vi "Set-UI-state.vi"(6 "State":T1, 8 "error in":errorcluster, 10 "Data ref. in":refnum<data-value>, 11 "UI ref. in":refnum<data-value>) -> (0 "error IO":errorcluster, 2 "Data ref.":refnum<data-value>, 3 "UI ref.":refnum<data-value>)   [LabVIEW 2013, in "CameraVision.lvlib" / "CV-UI.lvclass"]
doc: "This function deletes the data from the various GUI graphs and displays. This avoids interference with data from a previous acquisition."
uses:
  CV-UI.lvclass
  Main/Application-states.ctl
  Main/CV-Main.lvclass
  Control-names.ctl
  Main/Enqueue-modes.ctl
  Main/Main-actions.ctl
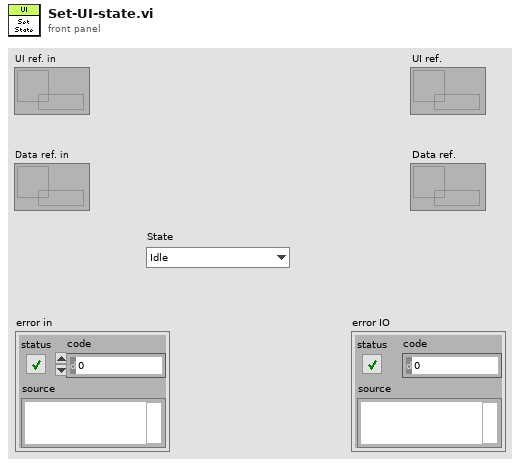
[diagram p1: front panel]
types:
  T1 = typedef "CameraVision.lvlib/CV-Main.lvclass/Application-states.ctl" = enum16{"Idle", "Initialized", "Configured", "Activated", "Started", "Stopped", "Reset", "Error", "Exited"}
  T2 = typedef "CameraVision.lvlib/CV-Main.lvclass/Enqueue-modes.ctl" = enum16{"Default", "Priority", "Flush"}
  T3 = typedef "CameraVision.lvlib/CV-UI.lvclass/Control-names.ctl" = enum16{"Start acquisition", "Activate", "Stop acquisition", "Settings type", "Load settings", "Save settings", "Import images", "Camera selector", "Image type selector", "Batch browser", "Image refresh", "Parameter tabs", "Displays", "Processing tabs", "Processing selector", "Map characteristic", "Show info", "Manual trigger"}
  T4 = typedef "CameraVision.lvlib/CV-Main.lvclass/Main-actions.ctl" = enum16{"Idle", "Initialize", "Load defaults", "Update settings", "Check settings", "Save settings", "Save settings with dialog", "Load settings", "Load data", "Activate", "Start", "Wait for start signal", "Acquire & process", "Iterate", "Stop", "Refresh display", "Refresh status", "View camera settings", "View grabber settings", "Exit"}
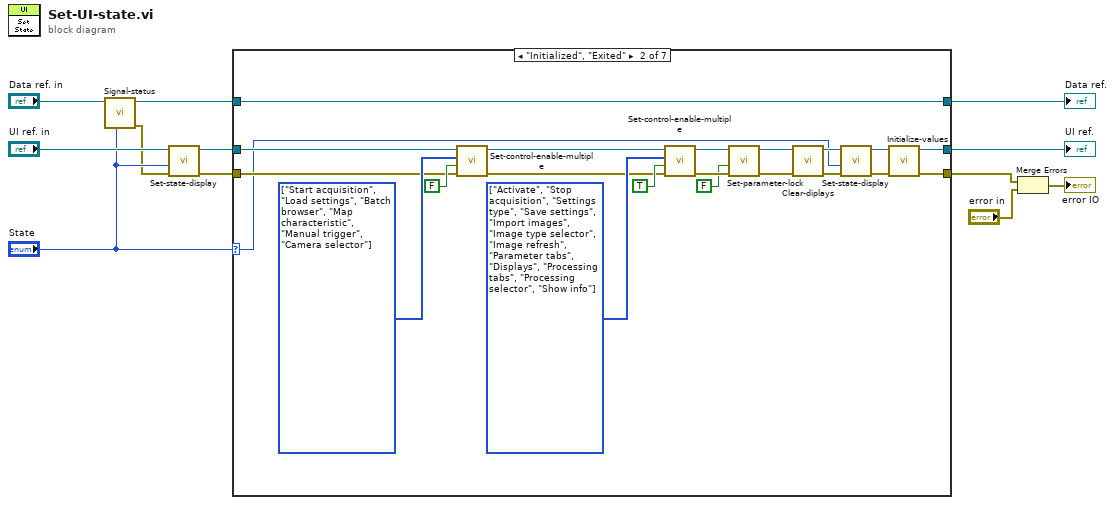
[diagram p0: block diagram]
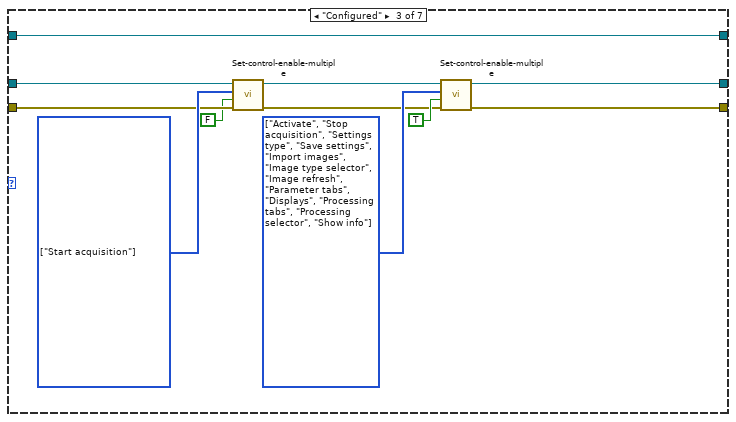
[diagram p3: hidden frame]
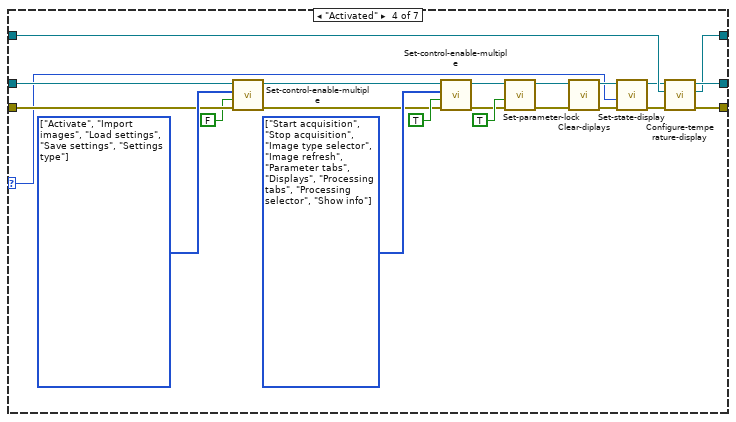
[diagram p4: hidden frame]
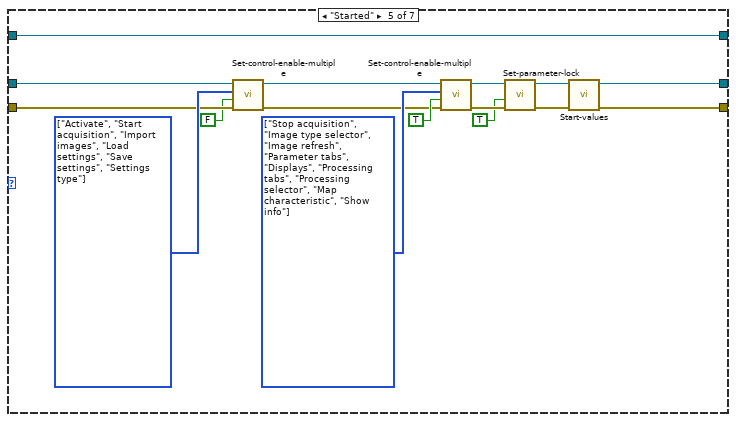
[diagram p5: hidden frame]
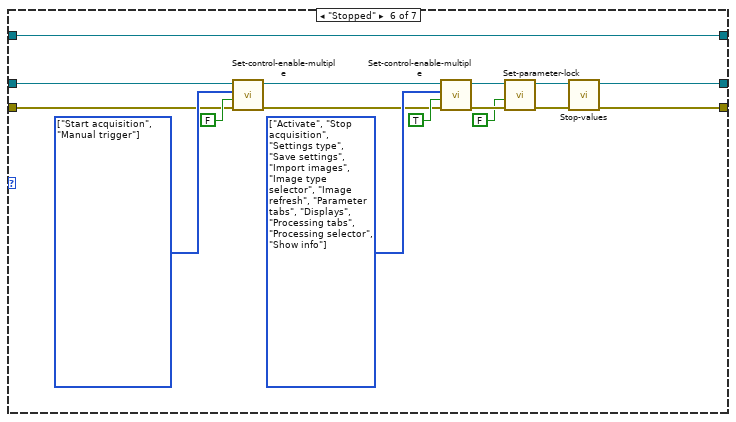
[diagram p6: hidden frame]
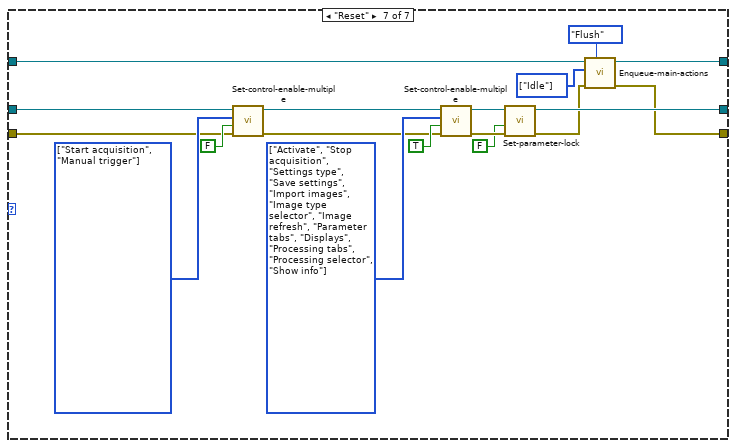
[diagram p7: hidden frame]
diagram:
  n1 = call "Signal-status.vi"("State"="State", "Data ref. in"="Data ref. in") -> ("error out"=w3:errorcluster, "Data ref."=w6:refnum<data-value>)  [unwired: 8 in]
  n2 = call "Set-state-display.vi"("error in"=w3, "State"="State", "UI ref. in"="UI ref. in") -> ("error IO"=w4:errorcluster, "UI ref."=w5:refnum<data-value>)  [unwired: 7 in]
  n3 = case shown="\"Initialized\", \"Exited\"" "State" {
    selector: "State" -> [_ w16 _ w48 _ _ _]
    tunnel: w4 -> [w14 w22 w45 w67 w83 w86 w108]
    tunnel: w5 -> [w15 w35 w46 w68 w84 w100 w118]
    tunnel: [w15 w23 w38 w56 w73 w91 w107] -> w10
    tunnel: [w14 w24 w39 w53 w74 w88 w104] -> w12
    tunnel: w6 -> [w13 w21 w37 w55 w70 w87 w109]
    tunnel: [w13 w21 w37 w54 w70 w87 w106] -> w7
    frame Default {
    }
    frame "Initialized", "Exited" {
      w33 = T3[] [enum."Activate", enum."Stop acquisition", enum."Settings type", enum."Save settings", enum."Import images", enum."Image type selector", enum."Image refresh", enum."Parameter tabs", enum."Displays", enum."Processing tabs", enum."Processing selector", enum."Show info"] items=["Start acquisition", "Activate", "Stop acquisition", "Settings type", "Load settings", "Save settings", "Import images", "Camera selector", "Image type selector", "Batch browser", "Image refresh", "Parameter tabs", "Displays", "Processing tabs", "Processing selector", "Map characteristic", "Show info", "Manual trigger"] ("Control names")
      w36 = T3[] [enum."Start acquisition", enum."Load settings", enum."Batch browser", enum."Map characteristic", enum."Manual trigger", enum."Camera selector"] items=["Start acquisition", "Activate", "Stop acquisition", "Settings type", "Load settings", "Save settings", "Import images", "Camera selector", "Image type selector", "Batch browser", "Image refresh", "Parameter tabs", "Displays", "Processing tabs", "Processing selector", "Map characteristic", "Show info", "Manual trigger"] ("Control names")
      n4 = call "Set-control-enable-multiple.vi"("error in (no error)"=w22, "Enable?"=FALSE, "Control names"=w36, "UI ref. in"=w35) -> ("error out"=w31:errorcluster, "UI ref."=w30:refnum<data-value>)  [unwired: 6 in]
      n5 = call "Set-control-enable-multiple.vi"("error in (no error)"=w31, "Enable?"=TRUE, "Control names"=w33, "UI ref. in"=w30) -> ("error out"=w28:errorcluster, "UI ref."=w29:refnum<data-value>)  [unwired: 6 in]
      n6 = call "Set-parameter-lock.vi"("error in (no error)"=w28, "Lock?"=FALSE, "UI ref. in"=w29) -> ("error out"=w25:errorcluster, "UI ref."=w26:refnum<data-value>)  [unwired: 7 in]
      n7 = call "Clear-diplays.vi"("error in"=w25, "UI ref. in"=w26) -> ("error IO"=w17:errorcluster, "UI ref."=w20:refnum<data-value>)  [unwired: 8 in]
      n8 = call "Set-state-display.vi"("error in"=w17, "State"=w16, "UI ref. in"=w20) -> ("error IO"=w18:errorcluster, "UI ref."=w19:refnum<data-value>)  [unwired: 7 in]
      n9 = call "Initialize-values.vi"("error in"=w18, "UI ref. in"=w19) -> ("error IO"=w24:errorcluster, "UI ref."=w23:refnum<data-value>)  [unwired: 8 in]
    }
    frame "Configured" {
      w43 = T3[] [enum."Activate", enum."Stop acquisition", enum."Settings type", enum."Save settings", enum."Import images", enum."Image type selector", enum."Image refresh", enum."Parameter tabs", enum."Displays", enum."Processing tabs", enum."Processing selector", enum."Show info"] items=["Start acquisition", "Activate", "Stop acquisition", "Settings type", "Load settings", "Save settings", "Import images", "Camera selector", "Image type selector", "Batch browser", "Image refresh", "Parameter tabs", "Displays", "Processing tabs", "Processing selector", "Map characteristic", "Show info", "Manual trigger"] ("Control names")
      w47 = T3[] [enum."Start acquisition"] items=["Start acquisition", "Activate", "Stop acquisition", "Settings type", "Load settings", "Save settings", "Import images", "Camera selector", "Image type selector", "Batch browser", "Image refresh", "Parameter tabs", "Displays", "Processing tabs", "Processing selector", "Map characteristic", "Show info", "Manual trigger"] ("Control names")
      n10 = call "Set-control-enable-multiple.vi"("error in (no error)"=w45, "Enable?"=FALSE, "Control names"=w47, "UI ref. in"=w46) -> ("error out"=w41:errorcluster, "UI ref."=w40:refnum<data-value>)  [unwired: 6 in]
      n11 = call "Set-control-enable-multiple.vi"("error in (no error)"=w41, "Enable?"=TRUE, "Control names"=w43, "UI ref. in"=w40) -> ("error out"=w39:errorcluster, "UI ref."=w38:refnum<data-value>)  [unwired: 6 in]
    }
    frame "Activated" {
      w65 = T3[] [enum."Start acquisition", enum."Stop acquisition", enum."Image type selector", enum."Image refresh", enum."Parameter tabs", enum."Displays", enum."Processing tabs", enum."Processing selector", enum."Show info"] items=["Start acquisition", "Activate", "Stop acquisition", "Settings type", "Load settings", "Save settings", "Import images", "Camera selector", "Image type selector", "Batch browser", "Image refresh", "Parameter tabs", "Displays", "Processing tabs", "Processing selector", "Map characteristic", "Show info", "Manual trigger"] ("Control names")
      w69 = T3[] [enum."Activate", enum."Import images", enum."Load settings", enum."Save settings", enum."Settings type"] items=["Start acquisition", "Activate", "Stop acquisition", "Settings type", "Load settings", "Save settings", "Import images", "Camera selector", "Image type selector", "Batch browser", "Image refresh", "Parameter tabs", "Displays", "Processing tabs", "Processing selector", "Map characteristic", "Show info", "Manual trigger"] ("Control names")
      n12 = call "Set-control-enable-multiple.vi"("error in (no error)"=w67, "Enable?"=FALSE, "Control names"=w69, "UI ref. in"=w68) -> ("error out"=w63:errorcluster, "UI ref."=w62:refnum<data-value>)  [unwired: 6 in]
      n13 = call "Set-control-enable-multiple.vi"("error in (no error)"=w63, "Enable?"=TRUE, "Control names"=w65, "UI ref. in"=w62) -> ("error out"=w59:errorcluster, "UI ref."=w60:refnum<data-value>)  [unwired: 6 in]
      n14 = call "Set-parameter-lock.vi"("error in (no error)"=w59, "Lock?"=TRUE, "UI ref. in"=w60) -> ("error out"=w58:errorcluster, "UI ref."=w57:refnum<data-value>)  [unwired: 7 in]
      n15 = call "Clear-diplays.vi"("error in"=w58, "UI ref. in"=w57) -> ("error IO"=w49:errorcluster, "UI ref."=w52:refnum<data-value>)  [unwired: 8 in]
      n16 = call "Set-state-display.vi"("error in"=w49, "State"=w48, "UI ref. in"=w52) -> ("error IO"=w50:errorcluster, "UI ref."=w51:refnum<data-value>)  [unwired: 7 in]
      n17 = call "Configure-temperature-display.vi"("error in"=w50, "Data ref. in"=w55, "UI ref. in"=w51) -> ("error IO"=w53:errorcluster, "Data ref."=w54:refnum<data-value>, "UI ref."=w56:refnum<data-value>)  [unwired: 6 in]
    }
    frame "Started" {
      w81 = T3[] [enum."Stop acquisition", enum."Image type selector", enum."Image refresh", enum."Parameter tabs", enum."Displays", enum."Processing tabs", enum."Processing selector", enum."Map characteristic", enum."Show info"] items=["Start acquisition", "Activate", "Stop acquisition", "Settings type", "Load settings", "Save settings", "Import images", "Camera selector", "Image type selector", "Batch browser", "Image refresh", "Parameter tabs", "Displays", "Processing tabs", "Processing selector", "Map characteristic", "Show info", "Manual trigger"] ("Control names")
      w85 = T3[] [enum."Activate", enum."Start acquisition", enum."Import images", enum."Load settings", enum."Save settings", enum."Settings type"] items=["Start acquisition", "Activate", "Stop acquisition", "Settings type", "Load settings", "Save settings", "Import images", "Camera selector", "Image type selector", "Batch browser", "Image refresh", "Parameter tabs", "Displays", "Processing tabs", "Processing selector", "Map characteristic", "Show info", "Manual trigger"] ("Control names")
      n18 = call "Set-control-enable-multiple.vi"("error in (no error)"=w83, "Enable?"=FALSE, "Control names"=w85, "UI ref. in"=w84) -> ("error out"=w79:errorcluster, "UI ref."=w78:refnum<data-value>)  [unwired: 6 in]
      n19 = call "Set-control-enable-multiple.vi"("error in (no error)"=w79, "Enable?"=TRUE, "Control names"=w81, "UI ref. in"=w78) -> ("error out"=w76:errorcluster, "UI ref."=w77:refnum<data-value>)  [unwired: 6 in]
      n20 = call "Set-parameter-lock.vi"("error in (no error)"=w76, "Lock?"=TRUE, "UI ref. in"=w77) -> ("error out"=w71:errorcluster, "UI ref."=w72:refnum<data-value>)  [unwired: 7 in]
      n21 = call "Start-values.vi"("error in"=w71, "UI ref. in"=w72) -> ("error IO"=w74:errorcluster, "UI ref."=w73:refnum<data-value>)  [unwired: 8 in]
    }
    frame "Stopped" {
      w98 = T3[] [enum."Activate", enum."Stop acquisition", enum."Settings type", enum."Save settings", enum."Import images", enum."Image type selector", enum."Image refresh", enum."Parameter tabs", enum."Displays", enum."Processing tabs", enum."Processing selector", enum."Show info"] items=["Start acquisition", "Activate", "Stop acquisition", "Settings type", "Load settings", "Save settings", "Import images", "Camera selector", "Image type selector", "Batch browser", "Image refresh", "Parameter tabs", "Displays", "Processing tabs", "Processing selector", "Map characteristic", "Show info", "Manual trigger"] ("Control names")
      w101 = T3[] [enum."Start acquisition", enum."Manual trigger"] items=["Start acquisition", "Activate", "Stop acquisition", "Settings type", "Load settings", "Save settings", "Import images", "Camera selector", "Image type selector", "Batch browser", "Image refresh", "Parameter tabs", "Displays", "Processing tabs", "Processing selector", "Map characteristic", "Show info", "Manual trigger"] ("Control names")
      n22 = call "Set-control-enable-multiple.vi"("error in (no error)"=w86, "Enable?"=FALSE, "Control names"=w101, "UI ref. in"=w100) -> ("error out"=w96:errorcluster, "UI ref."=w95:refnum<data-value>)  [unwired: 6 in]
      n23 = call "Set-control-enable-multiple.vi"("error in (no error)"=w96, "Enable?"=TRUE, "Control names"=w98, "UI ref. in"=w95) -> ("error out"=w93:errorcluster, "UI ref."=w94:refnum<data-value>)  [unwired: 6 in]
      n24 = call "Set-parameter-lock.vi"("error in (no error)"=w93, "Lock?"=FALSE, "UI ref. in"=w94) -> ("error out"=w89:errorcluster, "UI ref."=w90:refnum<data-value>)  [unwired: 7 in]
      n25 = call "Stop-values.vi"("error in"=w89, "UI ref. in"=w90) -> ("error IO"=w88:errorcluster, "UI ref."=w91:refnum<data-value>)  [unwired: 8 in]
    }
    frame "Reset" {
      w102 = T4[] [enum."Idle"] items=["Idle", "Initialize", "Load defaults", "Update settings", "Check settings", "Save settings", "Save settings with dialog", "Load settings", "Load data", "Activate", "Start", "Wait for start signal", "Acquire & process", "Iterate", "Stop", "Refresh display", "Refresh status", "View camera settings", "View grabber settings", "Exit"] ("State array")
      w116 = T3[] [enum."Activate", enum."Stop acquisition", enum."Settings type", enum."Save settings", enum."Import images", enum."Image type selector", enum."Image refresh", enum."Parameter tabs", enum."Displays", enum."Processing tabs", enum."Processing selector", enum."Show info"] items=["Start acquisition", "Activate", "Stop acquisition", "Settings type", "Load settings", "Save settings", "Import images", "Camera selector", "Image type selector", "Batch browser", "Image refresh", "Parameter tabs", "Displays", "Processing tabs", "Processing selector", "Map characteristic", "Show info", "Manual trigger"] ("Control names")
      w119 = T3[] [enum."Start acquisition", enum."Manual trigger"] items=["Start acquisition", "Activate", "Stop acquisition", "Settings type", "Load settings", "Save settings", "Import images", "Camera selector", "Image type selector", "Batch browser", "Image refresh", "Parameter tabs", "Displays", "Processing tabs", "Processing selector", "Map characteristic", "Show info", "Manual trigger"] ("Control names")
      n26 = call "Set-control-enable-multiple.vi"("error in (no error)"=w108, "Enable?"=FALSE, "Control names"=w119, "UI ref. in"=w118) -> ("error out"=w114:errorcluster, "UI ref."=w113:refnum<data-value>)  [unwired: 6 in]
      n27 = call "Set-control-enable-multiple.vi"("error in (no error)"=w114, "Enable?"=TRUE, "Control names"=w116, "UI ref. in"=w113) -> ("error out"=w111:errorcluster, "UI ref."=w112:refnum<data-value>)  [unwired: 6 in]
      n28 = call "Set-parameter-lock.vi"("error in (no error)"=w111, "Lock?"=FALSE, "UI ref. in"=w112) -> ("error out"=w105:errorcluster, "UI ref."=w107:refnum<data-value>)  [unwired: 7 in]
      n29 = call "Enqueue-main-actions.vi"("Enqueue mode"=Enqueue-modes."Flush", "error in (no error)"=w105, "State array"=w102, "Data ref. in"=w109) -> ("error out"=w104:errorcluster, "Data ref."=w106:refnum<data-value>)  [unwired: 5 in, 1 out]
    }
  }
  "UI ref." <- w10
  "Data ref." <- w7
  n30 = Merge Errors(w12, "error in") -> (→"error IO":errorcluster)
